vi "Receive Message.vi"(6 "priority":i32, 10 "IMediator in":refnum<class "IMediator.lvclass">, 11 "Message in":refnum<class "Message.lvclass">) -> (0 "error out":errorcluster, 2 "Actor out":refnum<class "Actor.lvclass">)   [LabVIEW 2020, in "MVA Framework.lvlib" / "IMediator.lvlib" / "IMediator.lvclass"]
doc: "This VI should be overriden ONLY if you are creating a proxy actor for remote transmission. If you are, override this VI to transmit the received message to a new destination, maintaining the given priority."
uses:
  IMediator.lvclass
  IMediator Messages/Publish Msg/Publish Msg.lvclass
  <vilib>/ActorFramework/Actor/Actor.lvclass
  <vilib>/ActorFramework/Message/Message.lvclass
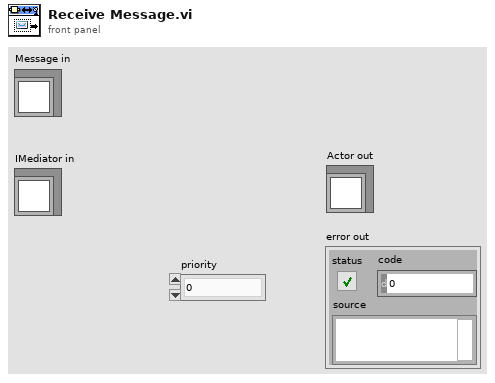
[diagram p1: front panel]
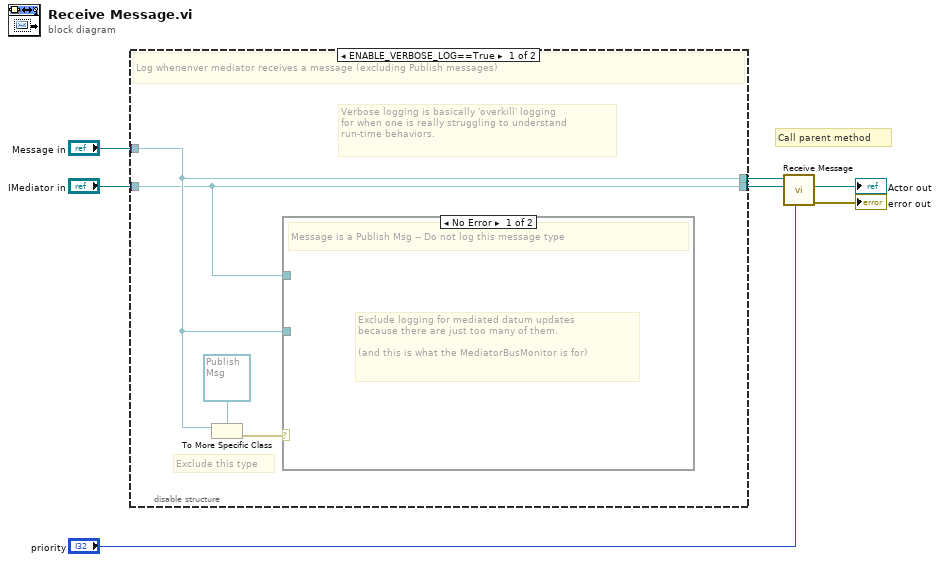
[diagram p0: block diagram]
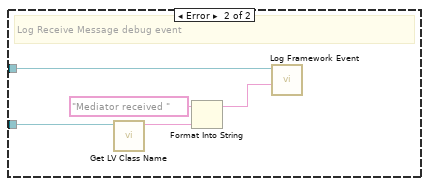
[diagram p2: hidden frame]
diagram:
  # "Call parent method"
  n1 = disable-structure shown="ENABLE_VERBOSE_LOG==True" {
    disable-tunnel: "Message in" -> [w11 w18]
    disable-tunnel: "IMediator in" -> [w10 w17]
    disable-tunnel: [w11 w18] -> w2
    disable-tunnel: [w10 w17] -> w1
    frame condition #0 {
      # "Verbose logging is basically 'overkill' logging\nfor when one is really struggling to understand\nrun-time behaviors."
      # "Exclude this type"
      # "Log whenenver mediator receives a message (excluding Publish messages)"
      n2 = To More Specific Class(target class=refnum<class "Publish Msg.lvclass"> refnum ("IMediator.lvlib:Publish Msg.lvclass"), reference=w11) -> (error out=w8:errorcluster)  [unwired: 1 in, 1 out]
      n3 = case shown="No Error" w8 {
        tunnel: w11 -> [_ w15]
        tunnel: w10 -> [_ w16]
        frame No Error {
          # "Exclude logging for mediated datum updates\nbecause there are just too many of them.\n\n(and this is what the MediatorBusMonitor is for)"
          # "Message is a Publish Msg -- Do not log this message type"
        }
        frame Error {
          # "Log Receive Message debug event"
          n4 = call <vilib>:"Get LV Class Name.vi"("object"=w15) -> ("class name"=w14:string)  [unwired: 9 in, 1 out]
          n5 = Format Into String(initial string="Mediator received ", w14) -> (resulting string=w12:string)  [unwired: 2 in, 1 out]
          n6 = call "Log Framework Event.vi"("Data To Log"=w12, "IMediator In"=w16) -> ()  [unwired: 9 in, 1 out]
        }
      }
    }
    frame condition #1 (active) {
      # "Remove all logging from this method at compile time"
    }
  }
  n7 = call-parent "Receive Message.vi"("priority"="priority", "Actor in"=w1, "Message in"=w2) -> ("error out"=→"error out":errorcluster, "Actor out"=→"Actor out":refnum<class "Actor.lvclass">)  [unwired: 7 in]
